vi "x Decode.vi"(2 "number":i32, 3 "x string":string) -> (0 "x string":string, 1 "number":i32)   [LabVIEW 2010, in "NI_Gmath.lvlib"]
uses:
  NI_Gmath.lvlib
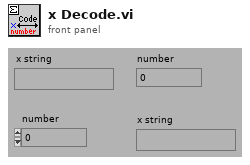
[diagram p1: front panel]
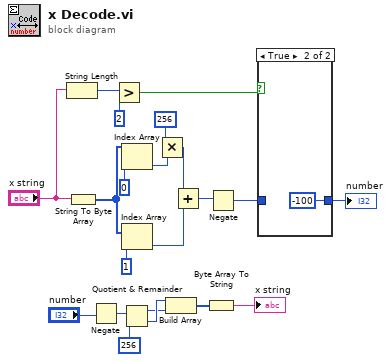
[diagram p0: block diagram]
diagram:
  n1 = String Length(string="x string") -> (length=w6:i32)
  n2 = String To Byte Array(string="x string") -> (unsigned byte array=w21:u8[])
  n3 = Negate(x="number") -> (-x=w13:i32)
  n4 = Greater?(x=w6, y=2) -> (0:w3:bool)
  n5 = Index Array(array=w21, index=0) -> (element=w18:u8)
  n6 = Index Array(array=w21, index=1) -> (element=w16:u8)
  n7 = Quotient & Remainder(x=w13, y=256) -> (x-y*floor(x/y)=w10:i32, floor(x/y)=w11:i32)
  n8 = Multiply(x=256, y=w18) -> (x*y=w15:i32)
  n9 = Build Array(w11, w10) -> (w9:i32[])
  n10 = Add(x=w15, y=w16) -> (x+y=w14:i32)
  n11 = Byte Array To String(unsigned byte array=w9) -> (string=→"x string":string)
  n12 = Negate(x=w14) -> (-x=w2:i32)
  n13 = case shown="True" w3 {
    tunnel: w2 -> [w22 _]
    tunnel: [w22 -100] -> w1
    frame False {
    }
    frame True {
    }
  }
  "number" <- w1
